vi "Destroy.vi"(8 "Error In":errorcluster, 11 "reference in":refnum<class "OD Entry.lvclass">) -> (0 "Error Out":errorcluster, 3 "reference out":refnum<class "OD Entry.lvclass">)   [LabVIEW 2020, in "Electronic Datasheet.lvlib" / "OD Entry.lvclass"]
uses:
  OD Entry.lvclass
  OD Sub-Entry/OD Sub-Entry.lvclass
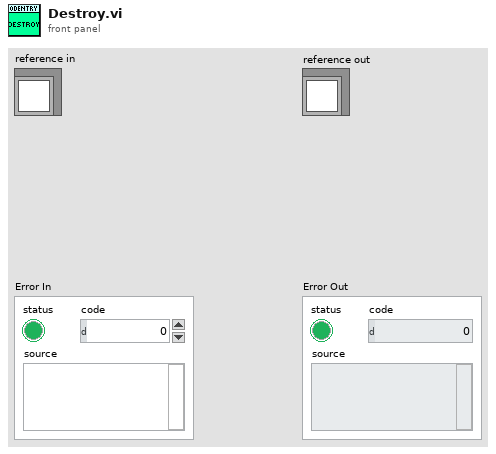
[diagram p1: front panel]
types:
  T1 = typedef "Electronic Datasheet.lvlib/OD Entry.lvclass/ObjectAttributes.ctl" = cluster{"Index":u16, "ObjectType":refnum<class "Object Type Base.lvclass">, "Denotation":string, "Count":u8, "ObjExtend":u8, "Label":string, "Description":string, "PDO Mapping Type":T2, "Sub-Entries":map{u8, refnum<class "OD Sub-Entry.lvclass">}}
  T2 = typedef "Electronic Datasheet.lvlib/PDO Mapping Type.ctl" = enum16{"no", "optional", "RPDO", "TPDO", "UNKNOWN"}
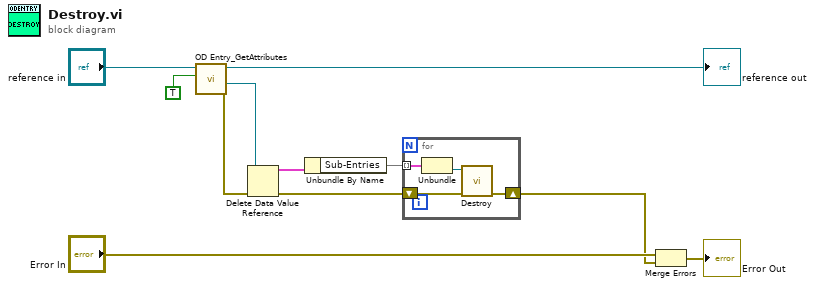
[diagram p0: block diagram]
diagram:
  n1 = call "OD Entry_GetAttributes.vi"("OnlyGetDvrReference(False)"=TRUE, "reference in"="reference in") -> ("Error Out"=w8:errorcluster, "DataRef"=w7:refnum<data-value>, "reference out"=→"reference out":refnum<class "OD Entry.lvclass">)  [unwired: 6 in, 1 out]
  n2 = Delete Data Value Reference(data value reference=w7, error in=w8) -> (data value=w4:T1, error out=w3:errorcluster)
  n3 = Unbundle By Name(w4) -> ("Sub-Entries"=w1:map{u8, refnum<class "OD Sub-Entry.lvclass">})
  n4 = for {
    tunnel: w1 -> [w15] mode=indexing
    shift-right: [w13] -> w2
    shift-left: w3 -> [w14]
    n5 = Unbundle(w15) -> ("OD Sub-Entry"=w12:refnum<class "OD Sub-Entry.lvclass">)  [unwired: 1 out]
    n6 = call-dynamic "Destroy.vi"("Error In"=w14, "reference in"=w12) -> ("Error Out"=w13:errorcluster)  [unwired: 8 in, 1 out]
  }
  n7 = Merge Errors("Error In", w2) -> (→"Error Out":errorcluster)
